vi "Get Marker Coordinates.vi"(8 "error in (no error)":errorcluster, 11 "GarphView in":refnum<class "GarphView.lvclass">) -> (0 "error out":errorcluster, 3 "GarphView out":refnum<class "GarphView.lvclass">)   [LabVIEW 2020, in "GarphView.lvlib" / "GarphView.lvclass"]
uses:
  GarphView.lvclass
  <vilib>/Utility/miscctls.llb/LVPoint32TypeDef.ctl
  GarphView.lvclass/GarphView.ctl
panel:
  out "XY":cluster{"X":dbl, "Y":dbl}
  in  "Coords":T1
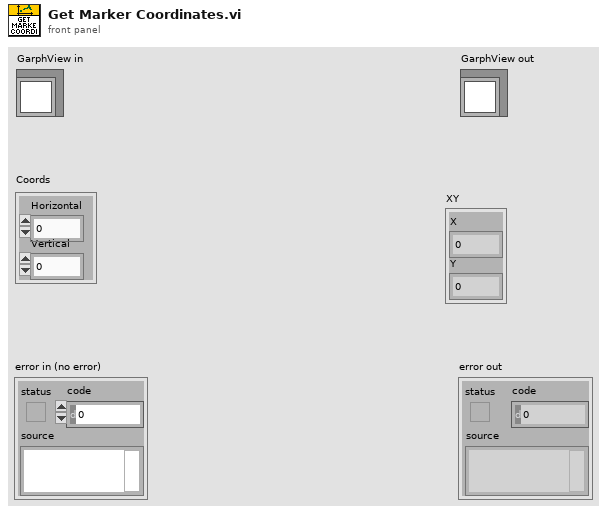
[diagram p1: front panel]
types:
  T1 = typedef "LVPoint32TypeDef.ctl" = cluster{"Horizontal":i32, "Vertical":i32}
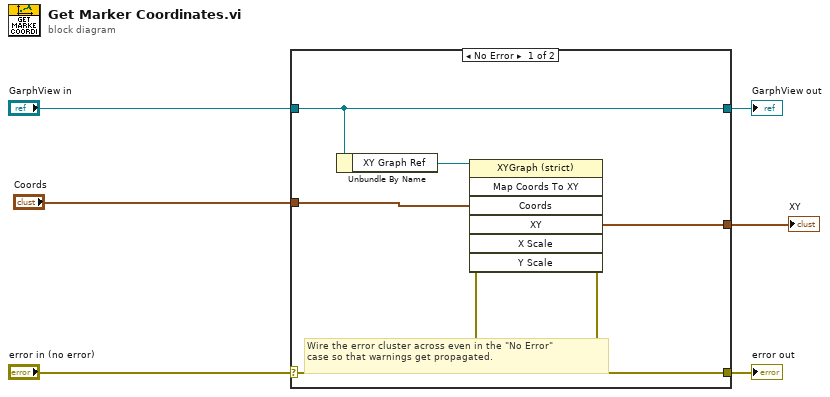
[diagram p0: block diagram]
diagram:
  n1 = case shown="No Error" "error in (no error)" {
    selector: "error in (no error)" -> [w8 w14]
    tunnel: [w7 w14] -> w5
    tunnel: [w11 w13] -> w3
    tunnel: "GarphView in" -> [w11 w13]
    tunnel: "Coords" -> [w12 _]
    tunnel: [w9 _] -> w1
    frame No Error {
      # "Wire the error cluster across even in the \"No Error\"\ncase so that warnings get propagated."
      n2 = Unbundle By Name(w11) -> ("XY Graph Ref"=w10:refnum<vi>)
      n3 = invoke class="XYGraph (strict)" method="Map Coords To XY"(reference=w10, error in=w8, "Coords"=w12) -> (error out=w7:errorcluster, "XY"=w9:cluster{"X":dbl, "Y":dbl})  [unwired: 4 in, 5 out]
    }
    frame Error {
    }
  }
  "error out" <- w5
  "GarphView out" <- w3
  "XY" <- w1
